vi "Select Signals.vi"(8 "Error In":errorcluster, 10 "Selection":cluster{"Type":T2, "Index(es)":i32[]}[](xcontrol), 11 "DATA IN":T1) -> (0 "Error Out":errorcluster, 2 "Fs":u32, 3 "Array":waveform(dbl)[](array[waveform]))   [LabVIEW 2017, in "Signal Selector.lvlib"]
uses:
  Signal Selector.lvlib
  Selection Folder/Selection.xctl
  PMU Buffer/Buffer DATA OUT ordered.ctl
  <vilib>/Analysis/baseanly.llb/Mean (DBL).vi
  <vilib>/Analysis/NI_AALPro.lvlib
  <vilib>/Analysis/NI_AALBase.lvlib
  PMU Buffer/PMU data buffer.lvlib
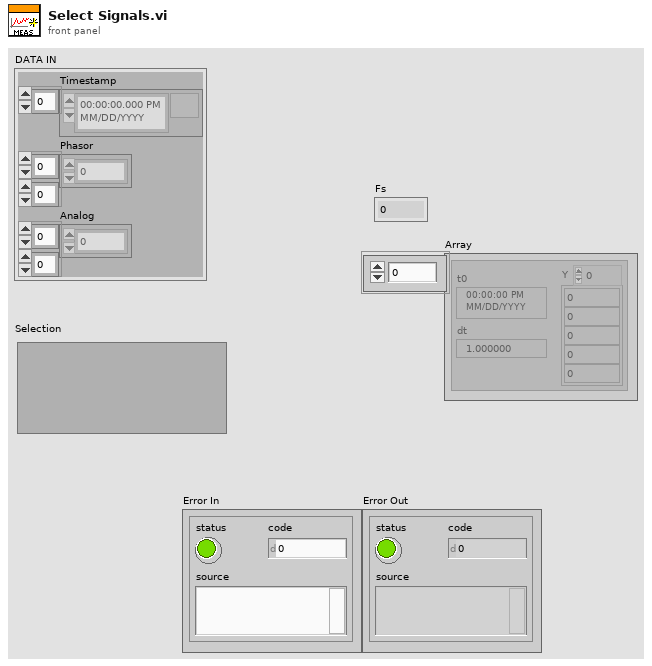
[diagram p1: front panel]
types:
  T1 = typedef "PMU data buffer.lvlib/Buffer DATA OUT ordered.ctl" = cluster{"Timestamp":timestamp[], "Phasor":csg[][], "Analog":sgl[][]}
  T2 = typedef "Selection.xctl/Signal types.ctl" = enum16{"Disable", "Frequency", "Phasor Mag", "Phasor Ang", "Angle Diff", "P", "Q"}
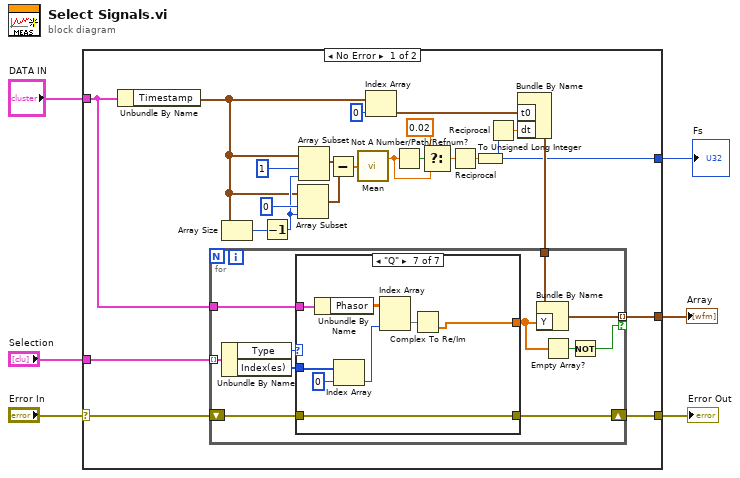
[diagram p0: block diagram]
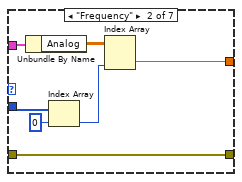
[diagram p3: hidden frame]
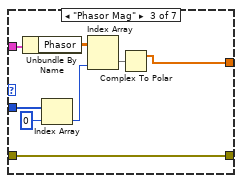
[diagram p4: hidden frame]
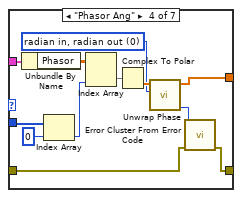
[diagram p5: hidden frame]
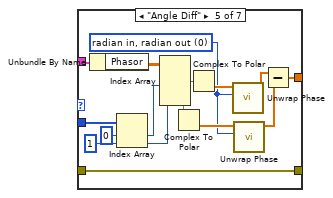
[diagram p6: hidden frame]
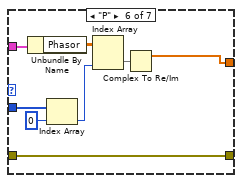
[diagram p7: hidden frame]
diagram:
  n1 = case shown="No Error" "Error In" {
    selector: "Error In" -> [w26 w101]
    tunnel: "Selection" -> [w29 _]
    tunnel: [w28 _] -> w6
    tunnel: [w25 w101] -> w4
    tunnel: [w8 _] -> w2
    tunnel: "DATA IN" -> [w16 _]
    frame No Error {
      n2 = Unbundle By Name(w16) -> ("Timestamp"=w13:timestamp[])
      n3 = Array Size(array=w13) -> (size(s)=w22:i32)
      n4 = Decrement(x=w22) -> (x-1=w21:i32)
      n5 = Array Subset(array=w13, index=0, length=w21) -> (w19:timestamp[])
      n6 = Array Subset(array=w13, index=1, length=w21) -> (w20:timestamp[])
      n7 = Subtract(x=w20, y=w19) -> (x-y=w18:dbl[])
      n8 = call-poly <vilib>:"Mean.vi"("X"=w18) -> ("mean"=w11:dbl)  [unwired: 1 out]
      n9 = Index Array(array=w13, index=0) -> (element=w14:timestamp)
      n10 = Not A Number/Path/Refnum?(number/path/refnum=w11) -> (NaN/Path/Refnum?=w12:bool)
      n11 = Select(t=0.02, s=w12, f=w11) -> (s? t:f=w9:dbl)
      n12 = Reciprocal(x=w9) -> (1/x=w17:dbl)
      n13 = To Unsigned Long Integer(number=w17) -> (unsigned 32bit integer=w8:u32)
      n14 = Reciprocal(x=w8) -> (1/x=w7:dbl)
      n15 = Bundle By Name("t0"=w14, "dt"=w7) -> (w27:waveform(dbl))  [unwired: 1 in]
      n16 = for {
        tunnel: w29 -> [w40] mode=indexing
        tunnel: w16 -> [w37]
        tunnel: [w36] -> w28 mode=indexing if=w30
        tunnel: w27 -> [w35]
        shift-right: [w33] -> w25
        shift-left: w26 -> [w34]
        n17 = Unbundle By Name(w40) -> ("Type"=w39:T2, "Index(es)"=w38:i32[])
        n18 = case shown="\"Q\"" w39 {
          tunnel: w38 -> [_ w46 w51 w60 w73 w87 w94]
          tunnel: w37 -> [_ w47 w56 w68 w84 w86 w96]
          tunnel: [_ w42 w53 w63 w75 w88 w95] -> w32
          tunnel: w34 -> [w41 w48 w52 w57 w74 w85 w93]
          tunnel: [w41 w48 w52 w62 w74 w85 w93] -> w33
          frame "Disable", Default {
          }
          frame "Frequency" {
            n19 = Unbundle By Name(w47) -> ("Analog"=w44:sgl[][])
            n20 = Index Array(array=w46, index=0) -> (element=w43:i32)
            n21 = Index Array(array=w44, index (col)=w43) -> (element=w42:sgl[])  [unwired: 1 in]
          }
          frame "Phasor Mag" {
            n22 = Unbundle By Name(w56) -> ("Phasor"=w55:csg[][])
            n23 = Index Array(array=w51, index=0) -> (element=w49:i32)
            n24 = Index Array(array=w55, index (col)=w49) -> (element=w54:csg[])  [unwired: 1 in]
            n25 = Complex To Polar(r * e^(i*theta)=w54) -> (r=w53:sgl[])  [unwired: 1 out]
          }
          frame "Phasor Ang" {
            w64 = 0 items=["radian in, radian out", "radian in, degree out", "degree in, degree out", "degree in, radian out"] ("phase unit")
            n26 = Unbundle By Name(w68) -> ("Phasor"=w67:csg[][])
            n27 = Index Array(array=w60, index=0) -> (element=w59:i32)
            n28 = Index Array(array=w67, index (col)=w59) -> (element=w66:csg[])  [unwired: 1 in]
            n29 = Complex To Polar(r * e^(i*theta)=w66) -> (theta=w65:sgl[])  [unwired: 1 out]
            n30 = call <vilib>:"Unwrap Phase.vi"("phase unit"=w64, "Phase"=w65) -> ("error"=w61:i32, "Unwrapped Phase"=w63:dbl[])  [unwired: 8 in]
            n31 = call <vilib>:"Error Cluster From Error Code.vi"("error in (no error)"=w57, "error code (0)"=w61) -> ("error out"=w62:errorcluster)  [unwired: 7 in]
          }
          frame "Angle Diff" {
            w78 = 0 items=["radian in, radian out", "radian in, degree out", "degree in, degree out", "degree in, radian out"] ("phase unit")
            n32 = Unbundle By Name(w84) -> ("Phasor"=w83:csg[][])
            n33 = Index Array(array=w73, index #1=0 ("index"), index #2=1 ("index")) -> (element #1=w70:i32, element #2=w69:i32)
            n34 = Index Array(array=w83, index (col) #1=w70, index (col) #2=w69) -> (element #1=w82:csg[], element #2=w81:csg[])  [unwired: 2 in]
            n35 = Complex To Polar(r * e^(i*theta)=w81) -> (theta=w80:sgl[])  [unwired: 1 out]
            n36 = Complex To Polar(r * e^(i*theta)=w82) -> (theta=w79:sgl[])  [unwired: 1 out]
            n37 = call <vilib>:"Unwrap Phase.vi"("phase unit"=w78, "Phase"=w79) -> ("Unwrapped Phase"=w77:dbl[])  [unwired: 8 in, 1 out]
            n38 = call <vilib>:"Unwrap Phase.vi"("phase unit"=w78, "Phase"=w80) -> ("Unwrapped Phase"=w76:dbl[])  [unwired: 8 in, 1 out]
            n39 = Subtract(x=w77, y=w76) -> (x-y=w75:dbl[])
          }
          frame "P" {
            n40 = Unbundle By Name(w86) -> ("Phasor"=w90:csg[][])
            n41 = Index Array(array=w87, index=0) -> (element=w92:i32)
            n42 = Index Array(array=w90, index (col)=w92) -> (element=w91:csg[])  [unwired: 1 in]
            n43 = Complex To Re/Im(x + iy=w91) -> (x=w88:sgl[])  [unwired: 1 out]
          }
          frame "Q" {
            n44 = Unbundle By Name(w96) -> ("Phasor"=w98:csg[][])
            n45 = Index Array(array=w94, index=0) -> (element=w100:i32)
            n46 = Index Array(array=w98, index (col)=w100) -> (element=w99:csg[])  [unwired: 1 in]
            n47 = Complex To Re/Im(x + iy=w99) -> (y=w95:sgl[])  [unwired: 1 out]
          }
        }
        n48 = Bundle By Name(cluster=w35, "Y"=w32) -> (w36:waveform(dbl))
        n49 = Empty Array?(array=w32) -> (empty?=w31:bool)
        n50 = Not(x=w31) -> (.not. x?=w30:bool)
      }
    }
    frame Error {
    }
  }
  "Array" <- w6
  "Error Out" <- w4
  "Fs" <- w2
